vi "Auto Loop 5.vi"(10 "auto #":u32, 11 "Call Context":T1) -> (0 "Loop 5 Value2":dbl, 1 "Loop 5 Value1":dbl, 2 "Loop 5 exit value":i32, 3 "Pneumatics SubState 5":T2)   [LabVIEW 2011]
uses:
  singleUseSubstate.ctl
  <vilib>/Rock Robotics/WPI/DriverStation/WPI_DriverStationDerivedRobotMode.ctl
  subStates.ctl
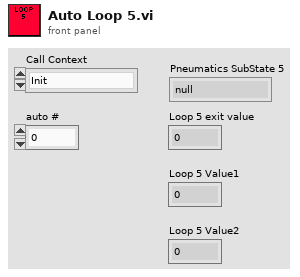
[diagram p1: front panel]
types:
  T1 = typedef "WPI_DriverStationDerivedRobotMode.ctl" = enum16{"Init", "Execute", "Stop"}
  T2 = typedef "singleUseSubstate.ctl" = enum16{"null", "wait", "shift", "shift high", "shift low", "bridge down", "bridge up", "extender in", "extender out", "extender toggle", "end"}
  T3 = typedef "subStates.ctl" = enum16{"null", "wait", "driver control", "auto", "manual override", "autoDrive", "hold position", "rotate", "end"}
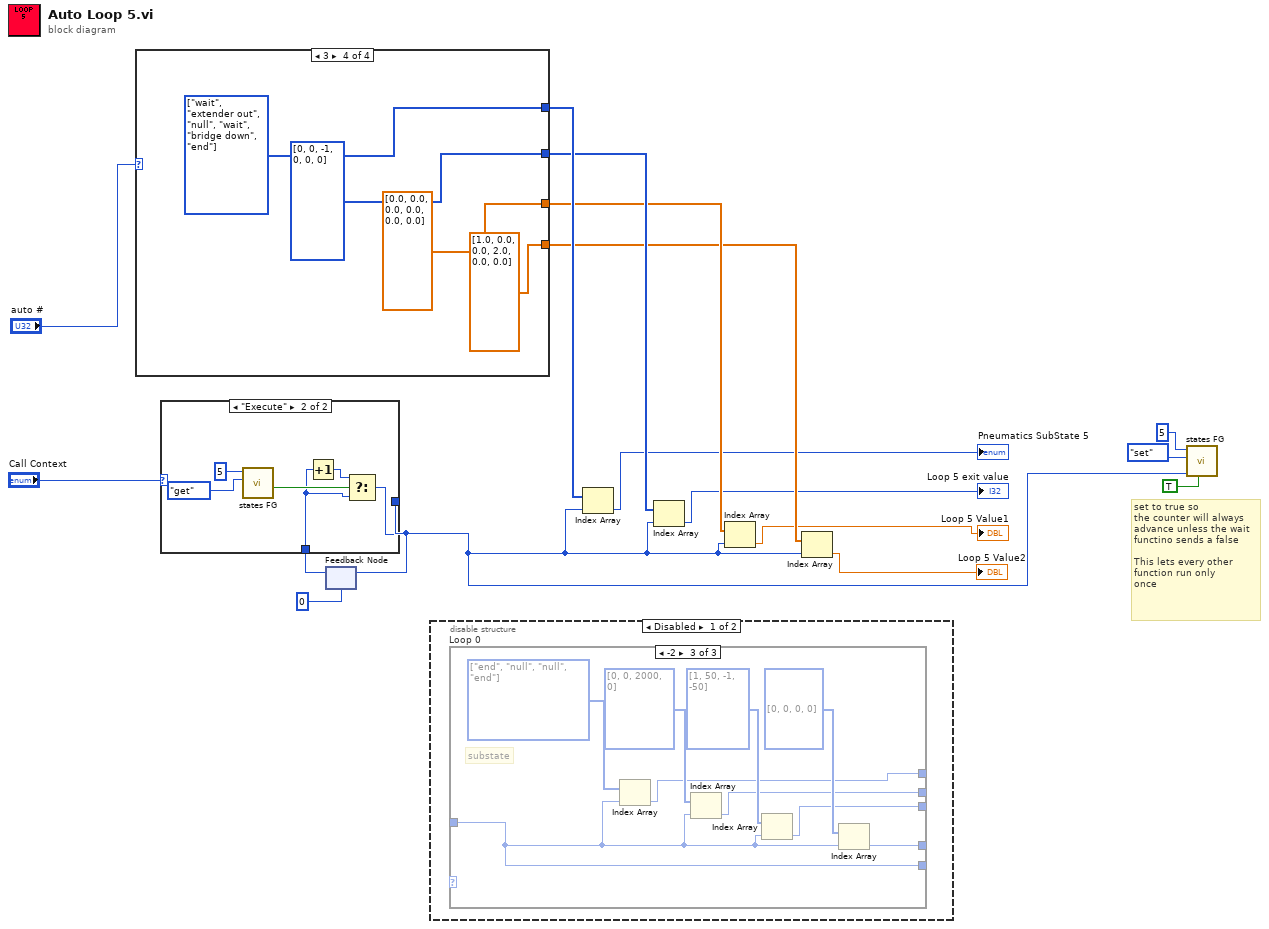
[diagram p0: block diagram]
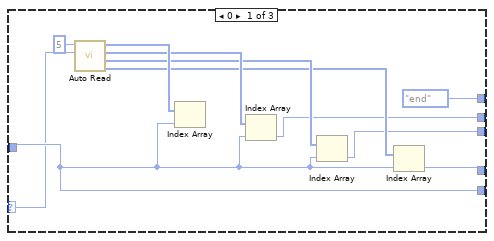
[diagram p2: hidden frame]
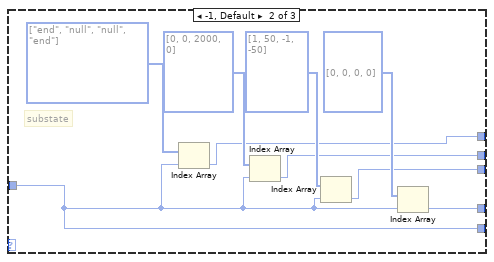
[diagram p3: hidden frame]
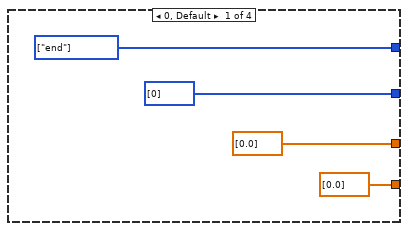
[diagram p5: hidden frame]
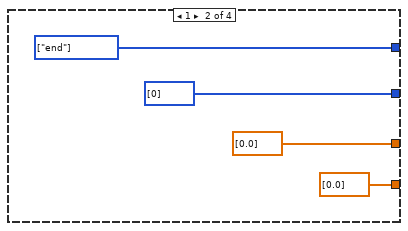
[diagram p6: hidden frame]
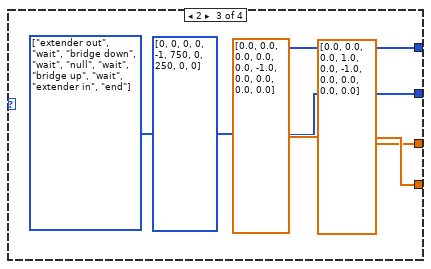
[diagram p7: hidden frame]
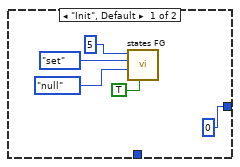
[diagram p8: hidden frame]
diagram:
  # "set to true so\nthe counter will always\nadvance unless the wait\nfunctino sends a false\n\nThis lets every other\nfunction run only\nonce"
  n1 = case shown="3" "auto #" {
    tunnel: [dbl[] [0.0] ("value2 array") dbl[] [0.0] ("value2 array") dbl[] [0.0, 0.0, 0.0, 1.0, 0.0, -1.0, 0.0, 0.0, 0.0, 0.0] ("value2 array") dbl[] [1.0, 0.0, 0.0, 2.0, 0.0, 0.0] ("value2 array")] -> w8
    tunnel: [dbl[] [0.0] ("value1 array") dbl[] [0.0] ("value1 array") dbl[] [0.0, 0.0, 0.0, 0.0, 0.0, -1.0, 0.0, 0.0, 0.0, 0.0] ("value1 array") dbl[] [0.0, 0.0, 0.0, 0.0, 0.0, 0.0] ("value1 array")] -> w9
    tunnel: [w18 w22 w26 w30] -> w11
    tunnel: [i32[] [0] ("exit value array") i32[] [0] ("exit value array") i32[] [0, 0, 0, 0, -1, 750, 0, 250, 0, 0] ("exit value array") i32[] [0, 0, -1, 0, 0, 0] ("exit value array")] -> w10
    frame 0, Default {
      w18 = T2[] [enum."end"] items=["null", "wait", "shift", "shift high", "shift low", "bridge down", "bridge up", "extender in", "extender out", "extender toggle", "end"] ("substate array")
    }
    frame 1 {
      w22 = T2[] [enum."end"] items=["null", "wait", "shift", "shift high", "shift low", "bridge down", "bridge up", "extender in", "extender out", "extender toggle", "end"] ("substate array")
    }
    frame 2 {
      w26 = T2[] [enum."extender out", enum."wait", enum."bridge down", enum."wait", enum."null", enum."wait", enum."bridge up", enum."wait", enum."extender in", enum."end"] items=["null", "wait", "shift", "shift high", "shift low", "bridge down", "bridge up", "extender in", "extender out", "extender toggle", "end"] ("substate array")
    }
    frame 3 {
      w30 = T2[] [enum."wait", enum."extender out", enum."null", enum."wait", enum."bridge down", enum."end"] items=["null", "wait", "shift", "shift high", "shift low", "bridge down", "bridge up", "extender in", "extender out", "extender toggle", "end"] ("substate array")
    }
  }
  n2 = feedback #1(0 ("Value1 2")) -> (w13:i32)
  n3 = case shown="\"Execute\"" "Call Context" {
    tunnel: [0 ("Value1 2") w42] -> w2
    tunnel: w13 -> [_ w39]
    frame "Init", Default {
      n4 = call "states FG.vi"("exit in"=TRUE, "subState in"=subStates."null", "menu (get)"=enum16{"set", "get"}."set", "Loop ID"=5) -> ()  [unwired: 4 in, 4 out]
    }
    frame "Execute" {
      n5 = call "states FG.vi"("menu (get)"=enum16{"set", "get"}."get", "Loop ID"=5) -> ("exit out"=w41:bool)  [unwired: 6 in, 3 out]
      n6 = Increment(x=w39) -> (x+1=w43:i32)
      n7 = Select(t=w43, s=w41, f=w39) -> (s? t:f=w42:i32)
    }
  }
  n8 = feedback-in #1(w2) -> ()
  n9 = disable-structure shown="Disabled" {
    frame Disabled {
      n10 = case "Loop 0" shown="-2" {
        selector: _ -> [w45 _ _]
        tunnel: _ -> [w53 w56 w65]
        tunnel: [w48 w59 w68] -> _
        tunnel: [w47 w58 w67] -> _
        tunnel: [w46 w57 w66] -> _
        tunnel: [w53 w56 w65] -> _
        tunnel: [singleUseSubstate."end" ("Pneumatics SubState 3") w55 w64] -> _
        frame 0 {
          n11 = call "Auto Read.vi"("auto#"=w45, "loop #"=5) -> ("value 2s"=w49:i32[], "value 1s"=w50:i32[], "exit values"=w51:i32[], "substates"=w52:T3[])  [unwired: 6 in]
          n12 = Index Array(array=w52, index=w53) -> ()  [unwired: 1 out]
          n13 = Index Array(array=w51, index=w53) -> (element=w48:i32)
          n14 = Index Array(array=w50, index=w53) -> (element=w47:i32)
          n15 = Index Array(array=w49, index=w53) -> (element=w46:i32)
        }
        frame -1, Default {
          w63 = T2[] [enum."end", enum."null", enum."null", enum."end"] items=["null", "wait", "shift", "shift high", "shift low", "bridge down", "bridge up", "extender in", "extender out", "extender toggle", "end"] ("SubState Array")
          # "val2"
          # "val1"
          # "exit"
          # "substate"
          n16 = Index Array(array=w63, index=w56) -> (element=w55:T2)
          n17 = Index Array(array=i32[] [0, 0, 2000, 0], index=w56) -> (element=w59:i32)
          n18 = Index Array(array=i32[] [1, 50, -1, -50], index=w56) -> (element=w58:i32)
          n19 = Index Array(array=i32[] [0, 0, 0, 0], index=w56) -> (element=w57:i32)
        }
        frame -2 {
          w72 = T2[] [enum."end", enum."null", enum."null", enum."end"] items=["null", "wait", "shift", "shift high", "shift low", "bridge down", "bridge up", "extender in", "extender out", "extender toggle", "end"] ("SubState Array")
          # "val2"
          # "val1"
          # "exit"
          # "substate"
          n20 = Index Array(array=w72, index=w65) -> (element=w64:T2)
          n21 = Index Array(array=i32[] [0, 0, 2000, 0], index=w65) -> (element=w68:i32)
          n22 = Index Array(array=i32[] [1, 50, -1, -50], index=w65) -> (element=w67:i32)
          n23 = Index Array(array=i32[] [0, 0, 0, 0], index=w65) -> (element=w66:i32)
        }
      }
    }
    frame Enabled {
    }
  }
  n24 = Index Array(array=w11, index=w2) -> (element=→"Pneumatics SubState 5":T2)
  n25 = Index Array(array=w10, index=w2) -> (element=→"Loop 5 exit value":i32)
  n26 = Index Array(array=w9, index=w2) -> (element=→"Loop 5 Value1":dbl)
  n27 = Index Array(array=w8, index=w2) -> (element=→"Loop 5 Value2":dbl)
  n28 = call "states FG.vi"("exit in"=TRUE, "state # in"=w2, "menu (get)"=enum16{"set", "get"}."set", "Loop ID"=5) -> ()  [unwired: 4 in, 4 out]
